vi "Double to Relative ns.vi"(3 "Double":dbl) -> (1 "Relative ns":i64)   [LabVIEW 2020, in "Vecto.lvlib"]
uses:
  Vecto.lvlib
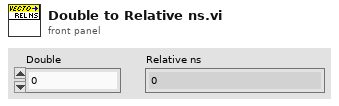
[diagram p1: front panel]
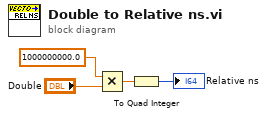
[diagram p0: block diagram]
diagram:
  n1 = Multiply(x=1000000000.0 ("y"), y="Double") -> (x*y=w3:dbl)
  n2 = To Quad Integer(1:w3) -> (0:→"Relative ns":i64)
